vi "addIntensity.vi"(8 "error in (no error)":errorcluster, 10 "lastMeasure":dbl, 11 "State in":refnum<class "State.lvclass">) -> (0 "error out":errorcluster, 3 "State out":refnum<class "State.lvclass">)   [LabVIEW 2016, in "State.lvclass"]
uses:
  State.lvclass
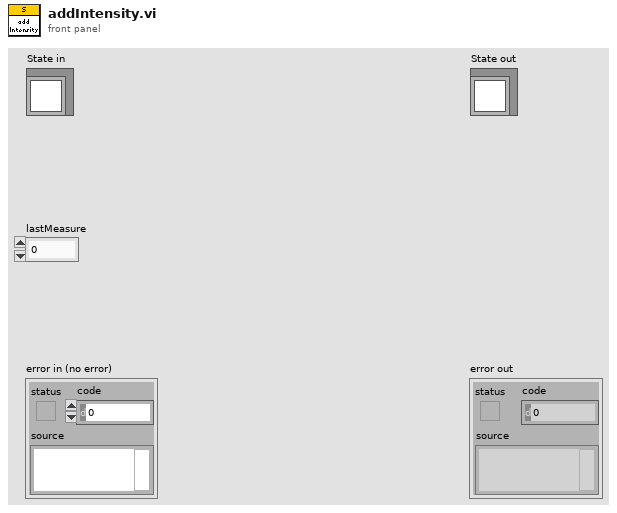
[diagram p1: front panel]
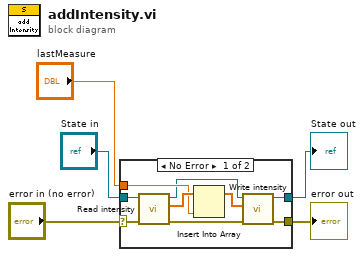
[diagram p0: block diagram]
diagram:
  n1 = case shown="No Error" "error in (no error)" {
    selector: "error in (no error)" -> [w13 w16]
    tunnel: [w7 w16] -> w4
    tunnel: [w6 w15] -> w2
    tunnel: "State in" -> [w14 w15]
    tunnel: "lastMeasure" -> [w11 _]
    frame No Error {
      n2 = call-dynamic "Read intensity.vi"("error in (no error)"=w13, "State in"=w14) -> ("error out"=w8:errorcluster, "intensity"=w12:dbl[], "State out"=w9:refnum<class "State.lvclass">)  [unwired: 7 in]
      n3 = Insert Into Array(array=w12, new element=w11) -> (w10:dbl[])  [unwired: 1 in]
      n4 = call-dynamic "Write intensity.vi"("error in (no error)"=w8, "intensity"=w10, "State in"=w9) -> ("error out"=w7:errorcluster, "State out"=w6:refnum<class "State.lvclass">)  [unwired: 7 in]
    }
    frame Error {
    }
  }
  "error out" <- w4
  "State out" <- w2
